vi "To HELP Line.vi"(8 "error in (no error)":errorcluster, 10 "Description":string, 11 "Name":string) -> (0 "error out":errorcluster, 3 "HELP line":string)   [LabVIEW 2020, in "Metrics.lvlib" / "Metric.lvclass"]
uses:
  Metric.lvclass
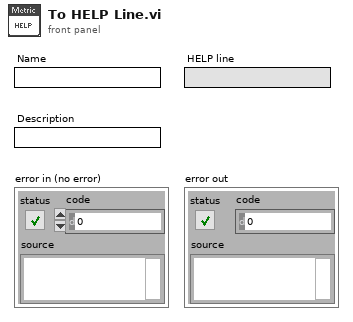
[diagram p1: front panel]
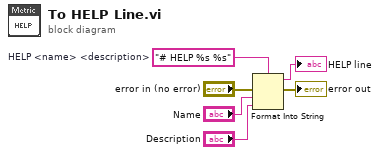
[diagram p0: block diagram]
diagram:
  w1 = "# HELP %s %s"  # HELP <name> <description>
  n1 = Format Into String(format string=w1, error in="error in (no error)", "Name", "Description") -> (resulting string=→"HELP line":string, error out=→"error out":errorcluster)  [unwired: 1 in]
